vi "VersaLaseGUItester.vi"() -> ()   [LabVIEW 2014]
uses:
  C:/Users/Avogadro/Desktop/VersaUSB/VersaUSB.dll
  VersaUSB.dll
panel:
  out "Blu Hrs":dbl
  out "Grn Hrs":dbl
  out "Red Hrs":dbl
  out "ne":i32
  out "e":i32
  in  "Blu Pow":dbl(slide) scale=0.0..100.0
  in  "Grn Pow":dbl(slide) scale=0.0..40.0
  in  "Blu On":bool
  in  "Grn On":bool
  out "Blu Temp":dbl
  out "Grn Temp":dbl
  in  "Red Pow":dbl(slide) scale=0.0..100.0
  in  "Red On":bool
  out "Red Temp":dbl
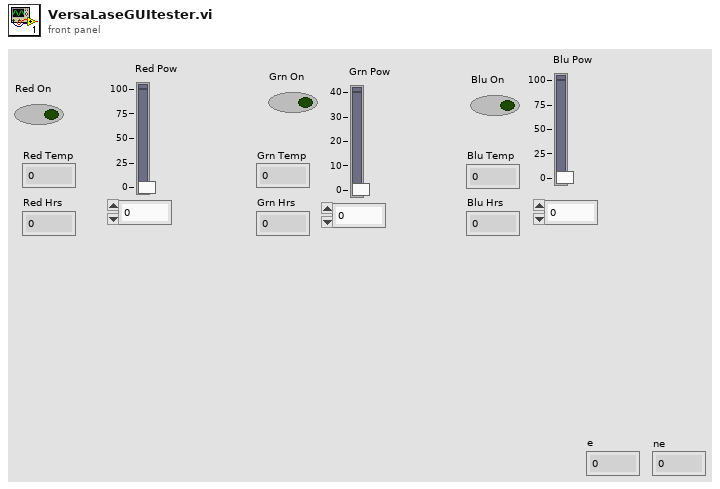
[diagram p1: front panel]
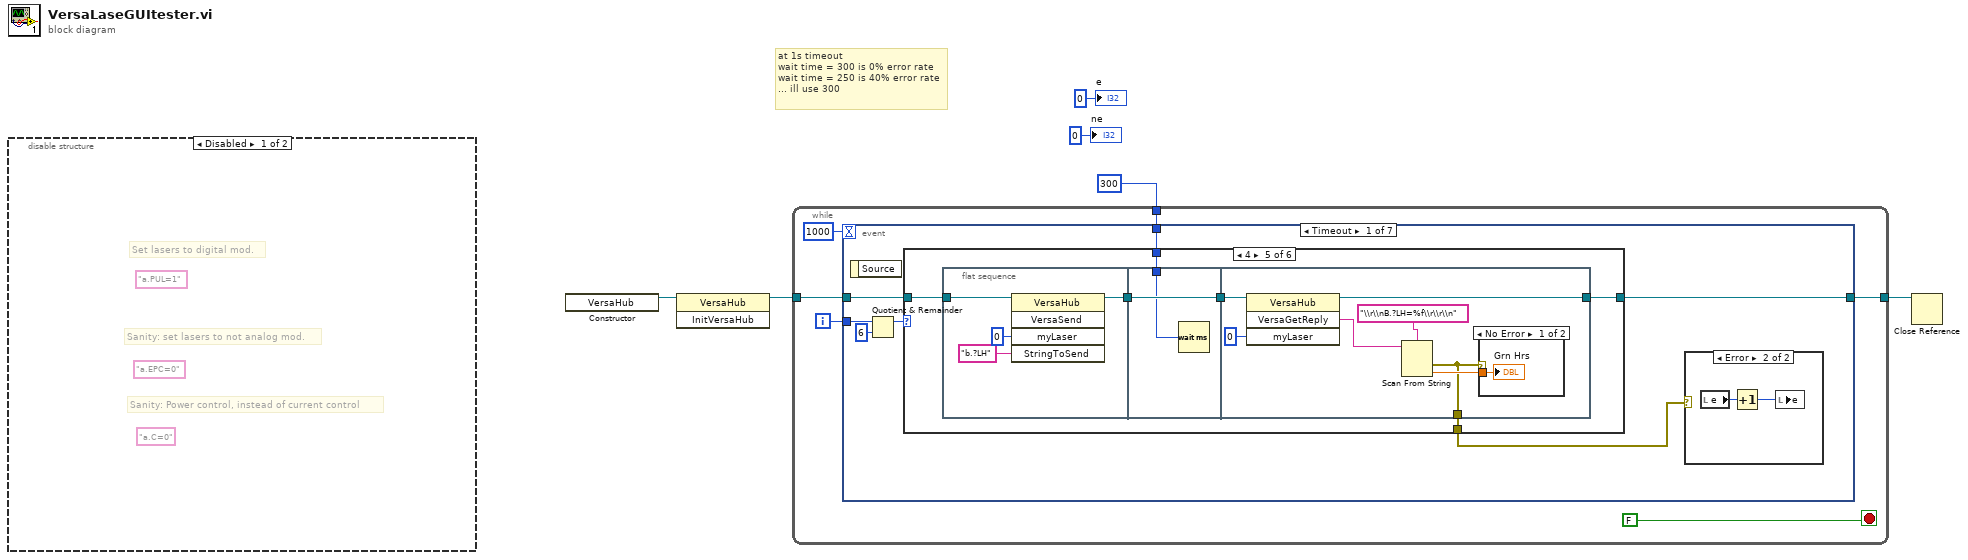
[diagram p0: block diagram]
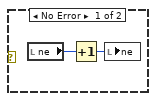
[diagram p3: hidden frame]
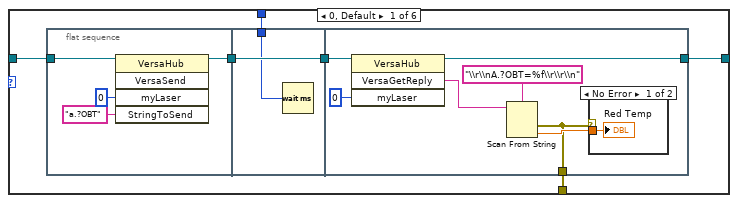
[diagram p4: hidden frame]
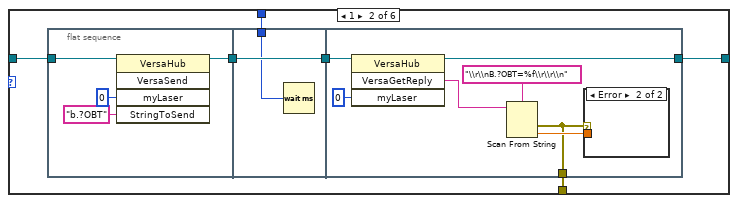
[diagram p6: hidden frame]
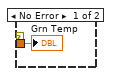
[diagram p7: hidden frame]
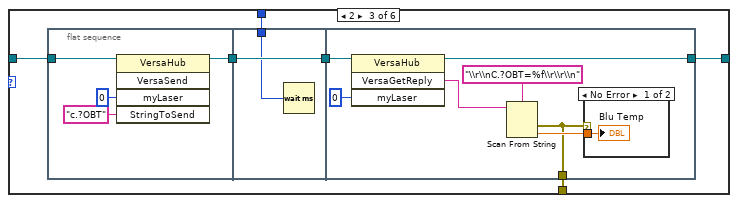
[diagram p8: hidden frame]
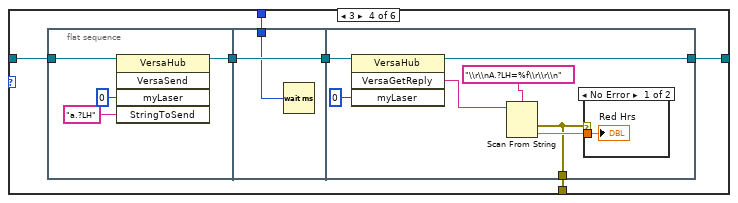
[diagram p10: hidden frame]
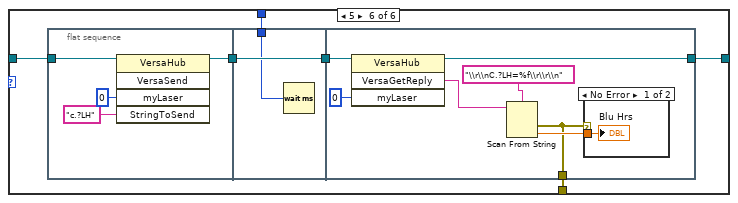
[diagram p13: hidden frame]
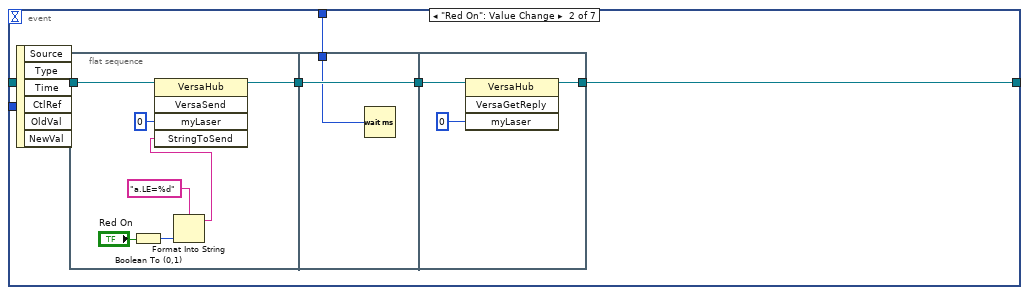
[diagram p15: hidden frame]
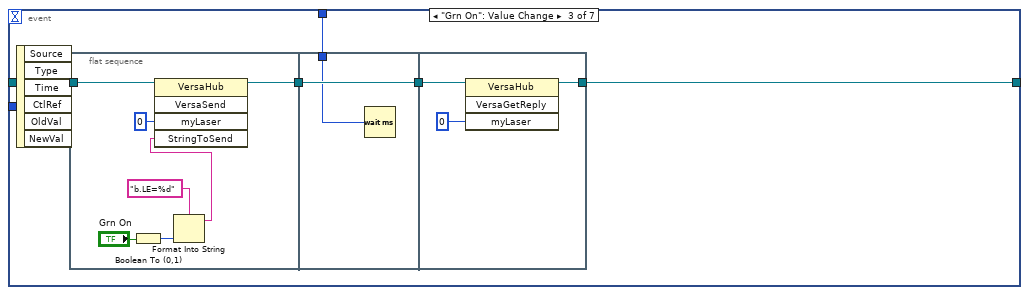
[diagram p16: hidden frame]
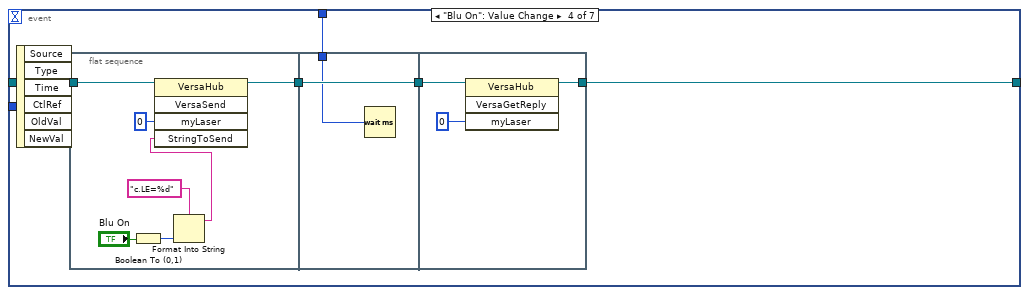
[diagram p17: hidden frame]
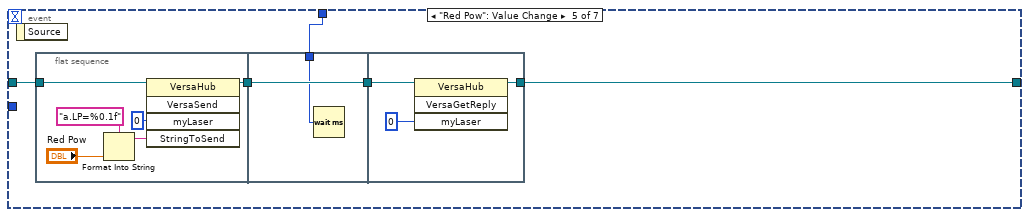
[diagram p18: hidden frame]
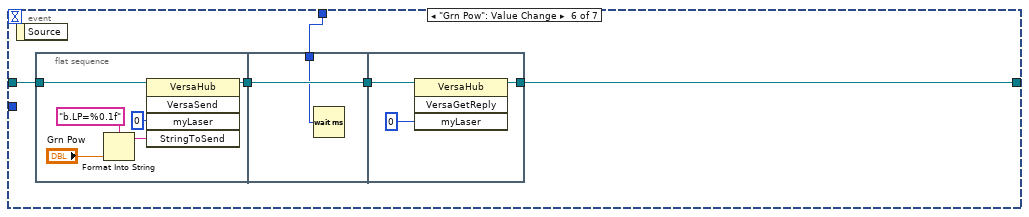
[diagram p19: hidden frame]
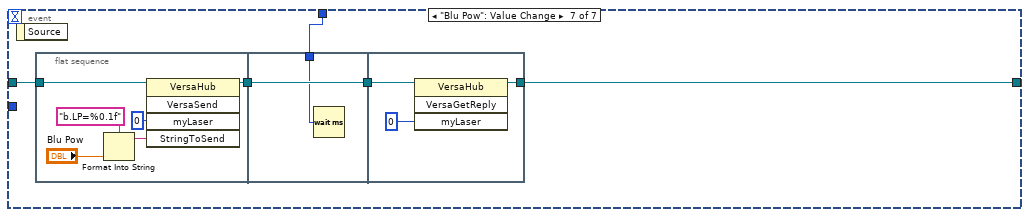
[diagram p20: hidden frame]
diagram:
  # "at 1s timeout\nwait time = 300 is 0% error rate\nwait time = 250 is 40% error rate\n... ill use 300"
  n1 = disable-structure shown="Disabled" {
    frame Disabled {
      (unwired) "a.C=0"
      (unwired) "a.EPC=0"
      (unwired) "a.PUL=1"
      # "Sanity: Power control, instead of current control"
      # "Sanity: set lasers to not analog mod."
      # "Set lasers to digital mod."
    }
    frame Enabled {
    }
  }
  n2 = constructor class="VersaHub"() -> (reference out=w5:refnum<k24>)  [unwired: 3 in, 2 out]
  n3 = invoke class="VersaHub" method="InitVersaHub"(reference=w5) -> (reference out=w6:refnum<k24>)  [unwired: 2 in, 2 out]
  n4 = while {
    tunnel: w6 -> [w12]
    tunnel: [w11] -> w4
    tunnel: u32 300 -> [w7]
    i -> [w8]
    stop <- FALSE stop-if-true
    n5 = event shown="[0] Timeout" {
      selector: _ -> [_ _ _ _ _ _ _]
      dyn-events: _ -> [_ _ _ _ _ _ _]
      timeout: 1000 -> [_ _ _ _ _ _ _]
      tunnel: w12 -> [w19 w148 w165 w182 w197 w213 w229]
      tunnel: [w13 w145 w162 w179 w196 w212 w228] -> w11
      tunnel: w8 -> [w18 _ _ _ _ _ _]
      tunnel: w7 -> [w15 w144 w161 w178 w195 w211 w227]
      event Timeout {
        n6 = event-data() -> ()  [unwired: 1 in, 1 out]
        n7 = Quotient & Remainder(x=w18, y=6) -> (x-y*floor(x/y)=w17:i32)  [unwired: 1 out]
        n8 = case shown="4" w17 {
          tunnel: w19 -> [w27 w47 w67 w87 w107 w127]
          tunnel: [w26 w46 w66 w86 w106 w126] -> w13
          tunnel: w15 -> [w25 w45 w65 w85 w105 w125]
          tunnel: [w24 w44 w64 w84 w104 w124] -> w14
          frame 0, Default {
            n9 = flat-sequence {
              tunnel: w27 -> [w33]
              tunnel: [w30] -> w29
              tunnel: w29 -> [w35]
              tunnel: [w35] -> w28
              tunnel: w25 -> [w34]
              tunnel: [w37] -> w26
              tunnel: w28 -> [w41]
              tunnel: [w36] -> w24
              frame #0 {
                n10 = invoke class="VersaHub" method="VersaSend"(reference=w33, "myLaser"=0, "StringToSend"="a.?OBT") -> (reference out=w30:refnum<k24>)  [unwired: 2 in, 4 out]
              }
              frame #1 {
                n11 = Wait (ms)(milliseconds to wait=w34) -> ()  [unwired: 1 out]
              }
              frame #2 {
                n12 = invoke class="VersaHub" method="VersaGetReply"(reference=w41, "myLaser"=0) -> (reference out=w37:refnum<k24>, "VersaGetReply"=w38:string)  [unwired: 2 in, 2 out]
                n13 = Scan From String(format string="\\r\\nA.?OBT=%f\\r\\r\\n", input string=w38) -> (error out=w36:errorcluster, output 1=w39:dbl)  [unwired: 3 in, 2 out]
                n14 = case shown="No Error" w36 {
                  tunnel: w39 -> [w43 _]
                  frame No Error {
                    "Red Temp" <- w43
                  }
                  frame Error {
                  }
                }
              }
            }
          }
          frame 1 {
            n15 = flat-sequence {
              tunnel: w47 -> [w53]
              tunnel: [w50] -> w49
              tunnel: w49 -> [w55]
              tunnel: [w55] -> w48
              tunnel: w45 -> [w54]
              tunnel: [w57] -> w46
              tunnel: w48 -> [w61]
              tunnel: [w56] -> w44
              frame #0 {
                n16 = invoke class="VersaHub" method="VersaSend"(reference=w53, "myLaser"=0, "StringToSend"="b.?OBT") -> (reference out=w50:refnum<k24>)  [unwired: 2 in, 4 out]
              }
              frame #1 {
                n17 = Wait (ms)(milliseconds to wait=w54) -> ()  [unwired: 1 out]
              }
              frame #2 {
                n18 = invoke class="VersaHub" method="VersaGetReply"(reference=w61, "myLaser"=0) -> (reference out=w57:refnum<k24>, "VersaGetReply"=w58:string)  [unwired: 2 in, 2 out]
                n19 = Scan From String(format string="\\r\\nB.?OBT=%f\\r\\r\\n", input string=w58) -> (error out=w56:errorcluster, output 1=w59:dbl)  [unwired: 3 in, 2 out]
                n20 = case shown="Error" w56 {
                  tunnel: w59 -> [w63 _]
                  frame No Error {
                    "Grn Temp" <- w63
                  }
                  frame Error {
                  }
                }
              }
            }
          }
          frame 2 {
            n21 = flat-sequence {
              tunnel: w67 -> [w73]
              tunnel: [w70] -> w69
              tunnel: w69 -> [w75]
              tunnel: [w75] -> w68
              tunnel: w65 -> [w74]
              tunnel: [w77] -> w66
              tunnel: w68 -> [w81]
              tunnel: [w76] -> w64
              frame #0 {
                n22 = invoke class="VersaHub" method="VersaSend"(reference=w73, "myLaser"=0, "StringToSend"="c.?OBT") -> (reference out=w70:refnum<k24>)  [unwired: 2 in, 4 out]
              }
              frame #1 {
                n23 = Wait (ms)(milliseconds to wait=w74) -> ()  [unwired: 1 out]
              }
              frame #2 {
                n24 = invoke class="VersaHub" method="VersaGetReply"(reference=w81, "myLaser"=0) -> (reference out=w77:refnum<k24>, "VersaGetReply"=w78:string)  [unwired: 2 in, 2 out]
                n25 = Scan From String(format string="\\r\\nC.?OBT=%f\\r\\r\\n", input string=w78) -> (error out=w76:errorcluster, output 1=w79:dbl)  [unwired: 3 in, 2 out]
                n26 = case shown="No Error" w76 {
                  tunnel: w79 -> [w83 _]
                  frame No Error {
                    "Blu Temp" <- w83
                  }
                  frame Error {
                  }
                }
              }
            }
          }
          frame 3 {
            n27 = flat-sequence {
              tunnel: w87 -> [w93]
              tunnel: [w90] -> w89
              tunnel: w89 -> [w95]
              tunnel: [w95] -> w88
              tunnel: w85 -> [w94]
              tunnel: [w97] -> w86
              tunnel: w88 -> [w101]
              tunnel: [w96] -> w84
              frame #0 {
                n28 = invoke class="VersaHub" method="VersaSend"(reference=w93, "myLaser"=0, "StringToSend"="a.?LH") -> (reference out=w90:refnum<k24>)  [unwired: 2 in, 4 out]
              }
              frame #1 {
                n29 = Wait (ms)(milliseconds to wait=w94) -> ()  [unwired: 1 out]
              }
              frame #2 {
                n30 = invoke class="VersaHub" method="VersaGetReply"(reference=w101, "myLaser"=0) -> (reference out=w97:refnum<k24>, "VersaGetReply"=w98:string)  [unwired: 2 in, 2 out]
                n31 = Scan From String(format string="\\r\\nA.?LH=%f\\r\\r\\n", input string=w98) -> (error out=w96:errorcluster, output 1=w99:dbl)  [unwired: 3 in, 2 out]
                n32 = case shown="No Error" w96 {
                  tunnel: w99 -> [w103 _]
                  frame No Error {
                    "Red Hrs" <- w103
                  }
                  frame Error {
                  }
                }
              }
            }
          }
          frame 4 {
            n33 = flat-sequence {
              tunnel: w107 -> [w113]
              tunnel: [w110] -> w109
              tunnel: w109 -> [w115]
              tunnel: [w115] -> w108
              tunnel: w105 -> [w114]
              tunnel: [w117] -> w106
              tunnel: w108 -> [w121]
              tunnel: [w116] -> w104
              frame #0 {
                n34 = invoke class="VersaHub" method="VersaSend"(reference=w113, "myLaser"=0, "StringToSend"="b.?LH") -> (reference out=w110:refnum<k24>)  [unwired: 2 in, 4 out]
              }
              frame #1 {
                n35 = Wait (ms)(milliseconds to wait=w114) -> ()  [unwired: 1 out]
              }
              frame #2 {
                n36 = invoke class="VersaHub" method="VersaGetReply"(reference=w121, "myLaser"=0) -> (reference out=w117:refnum<k24>, "VersaGetReply"=w118:string)  [unwired: 2 in, 2 out]
                n37 = Scan From String(format string="\\r\\nB.?LH=%f\\r\\r\\n", input string=w118) -> (error out=w116:errorcluster, output 1=w119:dbl)  [unwired: 3 in, 2 out]
                n38 = case shown="No Error" w116 {
                  tunnel: w119 -> [w123 _]
                  frame No Error {
                    "Grn Hrs" <- w123
                  }
                  frame Error {
                  }
                }
              }
            }
          }
          frame 5 {
            n39 = flat-sequence {
              tunnel: w127 -> [w133]
              tunnel: [w130] -> w129
              tunnel: w129 -> [w135]
              tunnel: [w135] -> w128
              tunnel: w125 -> [w134]
              tunnel: [w137] -> w126
              tunnel: w128 -> [w141]
              tunnel: [w136] -> w124
              frame #0 {
                n40 = invoke class="VersaHub" method="VersaSend"(reference=w133, "myLaser"=0, "StringToSend"="c.?LH") -> (reference out=w130:refnum<k24>)  [unwired: 2 in, 4 out]
              }
              frame #1 {
                n41 = Wait (ms)(milliseconds to wait=w134) -> ()  [unwired: 1 out]
              }
              frame #2 {
                n42 = invoke class="VersaHub" method="VersaGetReply"(reference=w141, "myLaser"=0) -> (reference out=w137:refnum<k24>, "VersaGetReply"=w138:string)  [unwired: 2 in, 2 out]
                n43 = Scan From String(format string="\\r\\nC.?LH=%f\\r\\r\\n", input string=w138) -> (error out=w136:errorcluster, output 1=w139:dbl)  [unwired: 3 in, 2 out]
                n44 = case shown="No Error" w136 {
                  tunnel: w139 -> [w143 _]
                  frame No Error {
                    "Blu Hrs" <- w143
                  }
                  frame Error {
                  }
                }
              }
            }
          }
        }
        n45 = case shown="Error" w14 {
          frame No Error {
            n46 = local read "ne"() -> (w21:i32)
            n47 = Increment(x=w21) -> (x+1=w20:i32)
            n48 = local write "ne"(w20) -> ()
          }
          frame Error {
            n49 = local read "e"() -> (w22:i32)
            n50 = Increment(x=w22) -> (x+1=w23:i32)
            n51 = local write "e"(w23) -> ()
          }
        }
      }
      event "Red On": Value Change {
        n52 = event-data() -> ()  [unwired: 1 in, 6 out]
        n53 = flat-sequence {
          tunnel: w148 -> [w155]
          tunnel: [w153] -> w147
          tunnel: w147 -> [w157]
          tunnel: [w157] -> w146
          tunnel: w144 -> [w156]
          tunnel: [w158] -> w145
          tunnel: w146 -> [w159]
          frame #0 {
            n54 = Boolean To (0,1)(Boolean="Red On") -> (0, 1=w151:i16)
            n55 = Format Into String(format string="a.LE=%d", w151) -> (resulting string=w149:string)  [unwired: 2 in, 1 out]
            n56 = invoke class="VersaHub" method="VersaSend"(reference=w155, "myLaser"=0, "StringToSend"=w149) -> (reference out=w153:refnum<k24>)  [unwired: 2 in, 4 out]
          }
          frame #1 {
            n57 = Wait (ms)(milliseconds to wait=w156) -> ()  [unwired: 1 out]
          }
          frame #2 {
            n58 = invoke class="VersaHub" method="VersaGetReply"(reference=w159, "myLaser"=0) -> (reference out=w158:refnum<k24>)  [unwired: 2 in, 3 out]
          }
        }
      }
      event "Grn On": Value Change {
        n59 = event-data() -> ()  [unwired: 1 in, 6 out]
        n60 = flat-sequence {
          tunnel: w165 -> [w172]
          tunnel: [w170] -> w164
          tunnel: w164 -> [w174]
          tunnel: [w174] -> w163
          tunnel: w161 -> [w173]
          tunnel: [w175] -> w162
          tunnel: w163 -> [w176]
          frame #0 {
            n61 = Boolean To (0,1)(Boolean="Grn On") -> (0, 1=w168:i16)
            n62 = Format Into String(format string="b.LE=%d", w168) -> (resulting string=w166:string)  [unwired: 2 in, 1 out]
            n63 = invoke class="VersaHub" method="VersaSend"(reference=w172, "myLaser"=0, "StringToSend"=w166) -> (reference out=w170:refnum<k24>)  [unwired: 2 in, 4 out]
          }
          frame #1 {
            n64 = Wait (ms)(milliseconds to wait=w173) -> ()  [unwired: 1 out]
          }
          frame #2 {
            n65 = invoke class="VersaHub" method="VersaGetReply"(reference=w176, "myLaser"=0) -> (reference out=w175:refnum<k24>)  [unwired: 2 in, 3 out]
          }
        }
      }
      event "Blu On": Value Change {
        n66 = event-data() -> ()  [unwired: 1 in, 6 out]
        n67 = flat-sequence {
          tunnel: w182 -> [w189]
          tunnel: [w187] -> w181
          tunnel: w181 -> [w191]
          tunnel: [w191] -> w180
          tunnel: w178 -> [w190]
          tunnel: [w192] -> w179
          tunnel: w180 -> [w193]
          frame #0 {
            n68 = Boolean To (0,1)(Boolean="Blu On") -> (0, 1=w185:i16)
            n69 = Format Into String(format string="c.LE=%d", w185) -> (resulting string=w183:string)  [unwired: 2 in, 1 out]
            n70 = invoke class="VersaHub" method="VersaSend"(reference=w189, "myLaser"=0, "StringToSend"=w183) -> (reference out=w187:refnum<k24>)  [unwired: 2 in, 4 out]
          }
          frame #1 {
            n71 = Wait (ms)(milliseconds to wait=w190) -> ()  [unwired: 1 out]
          }
          frame #2 {
            n72 = invoke class="VersaHub" method="VersaGetReply"(reference=w193, "myLaser"=0) -> (reference out=w192:refnum<k24>)  [unwired: 2 in, 3 out]
          }
        }
      }
      event "Red Pow": Value Change {
        n73 = event-data() -> ()  [unwired: 1 in, 1 out]
        n74 = flat-sequence {
          tunnel: w197 -> [w205]
          tunnel: [w203] -> w199
          tunnel: w199 -> [w207]
          tunnel: [w207] -> w198
          tunnel: w195 -> [w206]
          tunnel: [w208] -> w196
          tunnel: w198 -> [w209]
          frame #0 {
            n75 = Format Into String(format string="a.LP=%0.1f", "Red Pow") -> (resulting string=w200:string)  [unwired: 2 in, 1 out]
            n76 = invoke class="VersaHub" method="VersaSend"(reference=w205, "myLaser"=0, "StringToSend"=w200) -> (reference out=w203:refnum<k24>)  [unwired: 2 in, 4 out]
          }
          frame #1 {
            n77 = Wait (ms)(milliseconds to wait=w206) -> ()  [unwired: 1 out]
          }
          frame #2 {
            n78 = invoke class="VersaHub" method="VersaGetReply"(reference=w209, "myLaser"=0) -> (reference out=w208:refnum<k24>)  [unwired: 2 in, 3 out]
          }
        }
      }
      event "Grn Pow": Value Change {
        n79 = event-data() -> ()  [unwired: 1 in, 1 out]
        n80 = flat-sequence {
          tunnel: w213 -> [w221]
          tunnel: [w219] -> w215
          tunnel: w215 -> [w223]
          tunnel: [w223] -> w214
          tunnel: w211 -> [w222]
          tunnel: [w224] -> w212
          tunnel: w214 -> [w225]
          frame #0 {
            n81 = Format Into String(format string="b.LP=%0.1f", "Grn Pow") -> (resulting string=w216:string)  [unwired: 2 in, 1 out]
            n82 = invoke class="VersaHub" method="VersaSend"(reference=w221, "myLaser"=0, "StringToSend"=w216) -> (reference out=w219:refnum<k24>)  [unwired: 2 in, 4 out]
          }
          frame #1 {
            n83 = Wait (ms)(milliseconds to wait=w222) -> ()  [unwired: 1 out]
          }
          frame #2 {
            n84 = invoke class="VersaHub" method="VersaGetReply"(reference=w225, "myLaser"=0) -> (reference out=w224:refnum<k24>)  [unwired: 2 in, 3 out]
          }
        }
      }
      event "Blu Pow": Value Change {
        n85 = event-data() -> ()  [unwired: 1 in, 1 out]
        n86 = flat-sequence {
          tunnel: w229 -> [w237]
          tunnel: [w235] -> w231
          tunnel: w231 -> [w239]
          tunnel: [w239] -> w230
          tunnel: w227 -> [w238]
          tunnel: [w240] -> w228
          tunnel: w230 -> [w241]
          frame #0 {
            n87 = Format Into String(format string="b.LP=%0.1f", "Blu Pow") -> (resulting string=w232:string)  [unwired: 2 in, 1 out]
            n88 = invoke class="VersaHub" method="VersaSend"(reference=w237, "myLaser"=0, "StringToSend"=w232) -> (reference out=w235:refnum<k24>)  [unwired: 2 in, 4 out]
          }
          frame #1 {
            n89 = Wait (ms)(milliseconds to wait=w238) -> ()  [unwired: 1 out]
          }
          frame #2 {
            n90 = invoke class="VersaHub" method="VersaGetReply"(reference=w241, "myLaser"=0) -> (reference out=w240:refnum<k24>)  [unwired: 2 in, 3 out]
          }
        }
      }
    }
  }
  n91 = Close Reference(reference=w4) -> ()  [unwired: 1 in, 1 out]
  "e" <- 0 ("e")
  "ne" <- 0 ("ne")
